vi "Test_PT2.vi"() -> ()   [LabVIEW 2022 SP3, in "AnalogSignalProcessClass.lvclass"]
uses:
  AnalogSignalProcessClass.lvclass
  <vilib>/measure/NI_MABase.lvlib
panel:
  in  "T2":dbl
  out "XY Graph":cluster{dbl[], dbl[]}(graph)
  in  "sampling info":cluster{"Fs":dbl, "#s":dbl}={"Fs"=1000.0, "#s"=1000.0} {"Fs" format="%.2p"}
  in  "initialize":bool
  in  "T1":dbl
  in  "G":dbl
  in  "amplitude":dbl=1.0 format="%0.2p"
  in  "frequency":dbl=10.0 format="%0.2p"
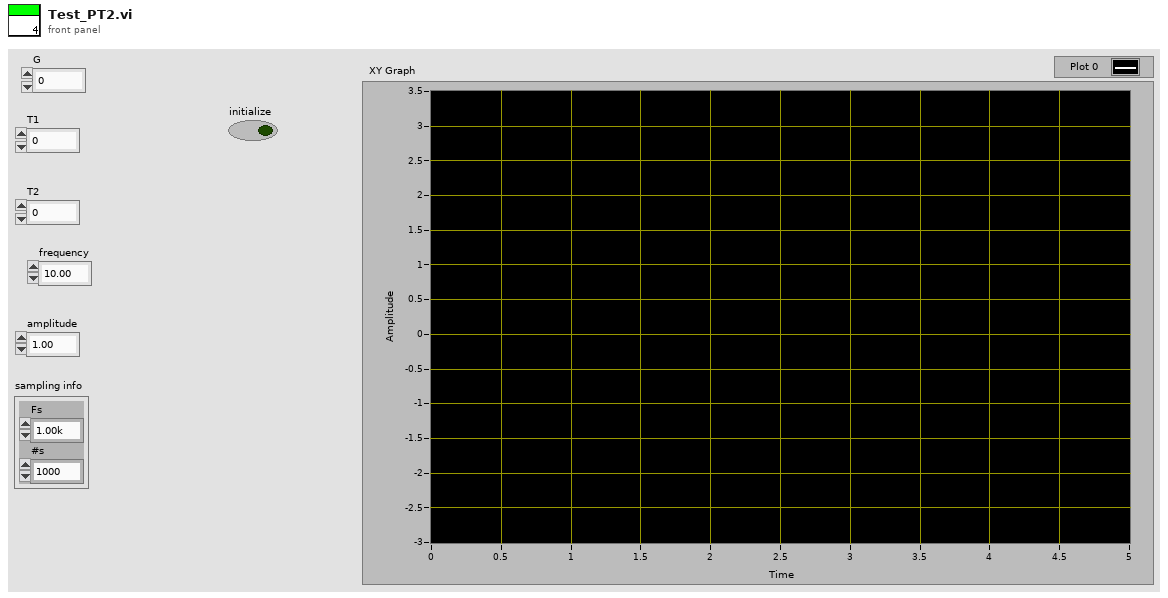
[diagram p1: front panel]
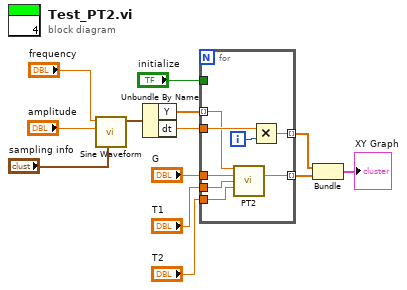
[diagram p0: block diagram]
diagram:
  n1 = call <vilib>:"Sine Waveform.vi"("sampling info"="sampling info", "amplitude"="amplitude", "frequency"="frequency") -> ("signal out"=w11:waveform(dbl))  [unwired: 7 in, 1 out]
  n2 = Unbundle By Name(w11) -> ("Y"=w10:dbl[], "dt"=w6:dbl)
  n3 = for {
    tunnel: w10 -> [w18] mode=indexing
    tunnel: "G" -> [w17]
    tunnel: "T1" -> [w16]
    tunnel: "initialize" -> [_]
    tunnel: w6 -> [w20]
    tunnel: [w19] -> w4 mode=indexing
    tunnel: "T2" -> [w15]
    tunnel: [w14] -> w2 mode=indexing
    i -> [w21]
    n4 = call "PT2.vi"("input u(k)"=w18, "G"=w17, "T1"=w16, "T2"=w15) -> ("output y(k)"=w14:dbl)  [unwired: 10 in, 1 out]
    n5 = Multiply(x=w20, y=w21) -> (x*y=w19:dbl)
  }
  n6 = Bundle(w4, w2) -> (→"XY Graph":cluster{dbl[], dbl[]})  [unwired: 1 in]
